vi "DHE_get_samplings.vi"(0 "fd in":i32, 11 "error in (no error)":errorcluster) -> (4 "fd out":i32, 6 "autoshutter":string, 15 "error out":errorcluster)   [LabVIEW 2016]
doc: "This VI closes the I/O interface with the instrument."
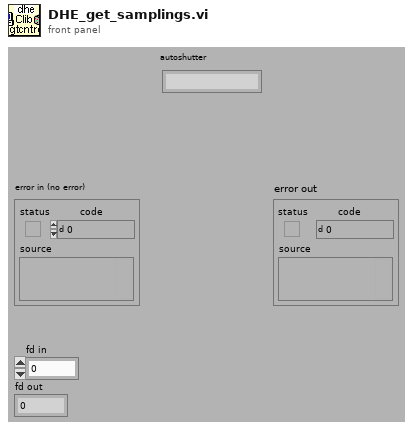
[diagram p1: front panel]
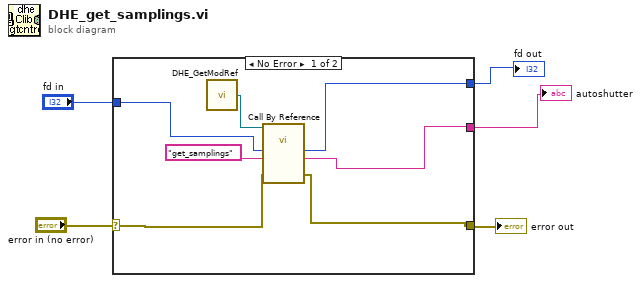
[diagram p0: block diagram]
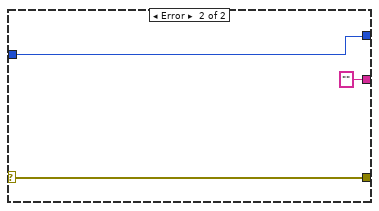
[diagram p2: hidden frame]
diagram:
  n1 = case shown="No Error" "error in (no error)" {
    selector: "error in (no error)" -> [w7 w15]
    tunnel: [w8 w15] -> w5
    tunnel: [w6 "" ("str result")] -> w1
    tunnel: "fd in" -> [w10 w14]
    tunnel: [w9 w14] -> w2
    frame No Error {
      n2 = call "DHE_GetModRef.vi"() -> ("DHE_ModRef"=w12:refnum<vi>)  [unwired: 9 out]
      n3 = call-by-ref "?"(reference=w12, "error in (no error)"=w7, "function"="get_samplings", "fd in"=w10) -> ("error out"=w8:errorcluster, "str result"=w6:string, "fd out"=w9:i32)  [unwired: 6 in, 3 out]
    }
    frame Error {
    }
  }
  "error out" <- w5
  "autoshutter" <- w1
  "fd out" <- w2
